vi "Ethernet IP Global GUIDs.vi"() -> ()   [LabVIEW 2011, in "Ethernet IP Custom Device Custom Device.lvlib"]
uses:
  Ethernet IP Custom Device Custom Device.lvlib
panel:
  in  "Sub":string="2F39BB52-EB64-6152-EE80-EBE234D27544"
  in  "Multiple":string="3B23EE4C-2EE3-F205-614C-CB8CFABA4D83"
  in  "Single":string="579C4C02-F42B-DFCB-13EA-649A60C99EE5"
  in  "Import Info and Unconfigured":string="CDFD8CDF-FF09-4A09-8179-2A3DE26A5307"
  in  "IO Folder":string="34030416-2576-DFCF-6977-C3963092562C"
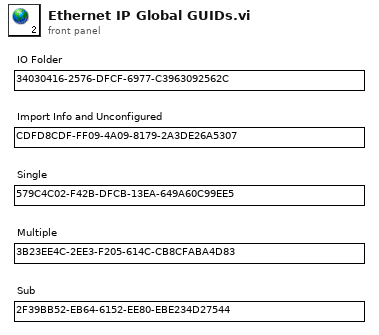
[diagram p1: front panel]
diagram:
